vi "ConfigureDriverProfiles.vi"(6 "Apply New Setpoint":bool, 8 "New Setpoints":dbl[](array[numeric]), 9 "Selected Driver":i32, 10 "Setpoint Save Location":path, 11 "Driver Profile Names":string[](array[string])) -> (3 "Current Setpoints":dbl[](array[numeric]))   [LabVIEW 2019]
doc: "This VI allows the user to change driver profile settings from the FRC 4265 dashboard and save them to the roboRIO."
uses:
  <vilib>/Utility/xml.llb/Write to XML File(string).vi
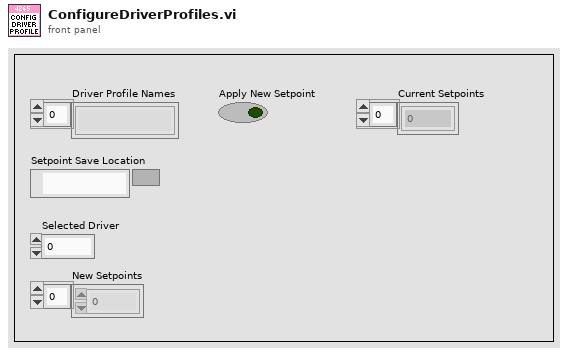
[diagram p1: front panel]
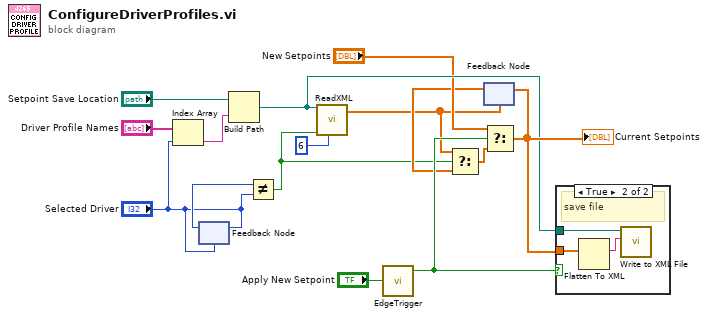
[diagram p0: block diagram]
diagram:
  n1 = Index Array(array="Driver Profile Names", index="Selected Driver") -> (element=w10:string)
  n2 = feedback-in #1("Selected Driver") -> ()
  n3 = feedback #1("Selected Driver") -> (w8:i32)
  n4 = Build Path(base path="Setpoint Save Location", name or relative path=w10) -> (appended path=w9:path)
  n5 = Not Equal?(x=w8, y="Selected Driver") -> (x != y?=w2:bool)
  n6 = call "ReadXML.vi"("Default Number of Elements"=6, "Reinit"=w2, "File Path (.xml)"=w9) -> ("Data"=w1:dbl[])  [unwired: 7 in, 1 out]
  n7 = call "EdgeTrigger.vi"("Input Signal"="Apply New Setpoint") -> ("Rising Edge Trigger"=w14:bool)  [unwired: 2 out]
  n8 = feedback #2(w1) -> (w3:dbl[])
  n9 = Select(t=w1, s=w2, f=w3) -> (s? t:f=w4:dbl[])
  n10 = Select(t="New Setpoints", s=w14, f=w4) -> (s? t:f=w15:dbl[])
  "Current Setpoints" <- w15
  n11 = feedback-in #2(w15) -> ()
  n12 = case shown="True" w14 {
    tunnel: w15 -> [_ w17]
    tunnel: w9 -> [_ w16]
    frame False {
    }
    frame True {
      # "save file"
      n13 = Flatten To XML(anything=w17) -> (xml string=w18:string)
      n14 = call-poly <vilib>:"Write to XML File.vi"("XML Input"=w18, "XML File Path"=w16) -> ()  [unwired: 7 in, 3 out]
    }
  }
